vi "verify unique parameter in range - SET.vi"(8 "error in (no error)":errorcluster, 9 "value":dbl, 10 "parameter name":string, 11 "Simulated_CCD_Camera in":refnum<class "Sim_Ixon_Ultra.lvclass">) -> (0 "error out":errorcluster, 3 "Simulated_CCD_Camera out":refnum<class "Sim_Ixon_Ultra.lvclass">)   [LabVIEW 2018, in "Sim_Ixon_Ultra.lvclass"]
uses:
  Sim_Ixon_Ultra.lvclass
  <vilib>/ErrorRing/Error Ring.xnode
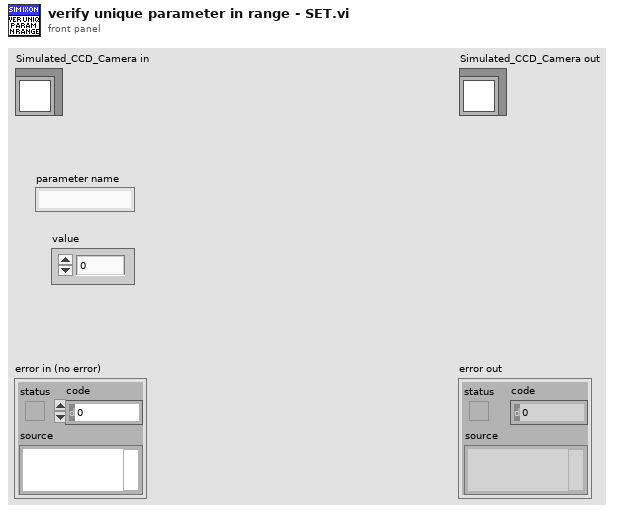
[diagram p1: front panel]
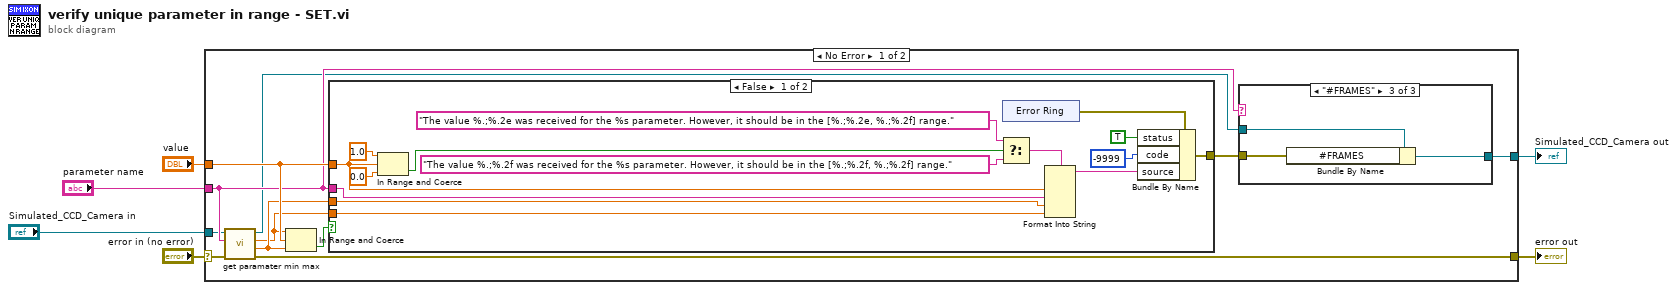
[diagram p0: block diagram]
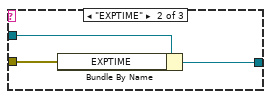
[diagram p3: hidden frame]
diagram:
  n1 = case shown="No Error" "error in (no error)" {
    selector: "error in (no error)" -> [w11 w42]
    tunnel: [w7 w42] -> w5
    tunnel: [w8 w41] -> w4
    tunnel: "Simulated_CCD_Camera in" -> [w12 w41]
    tunnel: "value" -> [w16 _]
    tunnel: "parameter name" -> [w15 _]
    frame No Error {
      n2 = call "get paramater min max.vi"("error in (no error)"=w11, "parameter name"=w15, "Simulated Camera in"=w12) -> ("error out"=w7:errorcluster, "min"=w14:dbl, "max"=w13:dbl, "Simulated Camera out"=w10:refnum<class "Sim_Ixon_Ultra.lvclass">)  [unwired: 5 in]
      n3 = In Range and Coerce(upper limit=w13, x=w16, lower limit=w14) -> (In Range?=w17:bool)  [unwired: 1 out]
      n4 = case shown="False" w17 {
        tunnel: w15 -> [w26 _]
        tunnel: w16 -> [w31 _]
        tunnel: w14 -> [w35 _]
        tunnel: w13 -> [w34 _]
        tunnel: [w25 _] -> w9
        frame False {
          n5 = In Range and Coerce(upper limit=1.0, x=w31, lower limit=0.0 ("upper limit")) -> (In Range?=w30:bool)  [unwired: 1 out]
          n6 = Select(t="The value %.;%.2e was received for the %s parameter. However, it should be in the [%.;%.2e, %.;%.2f] range." ("string"), s=w30, f="The value %.;%.2f was received for the %s parameter. However, it should be in the [%.;%.2f, %.;%.2f] range." ("string")) -> (s? t:f=w27:string)
          n7 = xnode "Error Ring"() -> ("error out"=w39:errorcluster)
          n8 = Format Into String(format string=w27, w31, w26, w35, w34) -> (resulting string=w36:string)  [unwired: 2 in, 1 out]
          n9 = Bundle By Name(cluster=w39, "status"=TRUE, "code"=-9999, "source"=w36) -> (w25:errorcluster)
        }
        frame True {
        }
      }
      n10 = case shown="\"#FRAMES\"" w15 {
        tunnel: w10 -> [w18 w21 w24]
        tunnel: [w18 w20 w23] -> w8
        tunnel: w9 -> [_ w19 w22]
        frame "False", Default {
        }
        frame "EXPTIME" {
          n11 = Bundle By Name(cluster=w21, "EXPTIME"=w19) -> (w20:refnum<class "Sim_Ixon_Ultra.lvclass">)
        }
        frame "#FRAMES" {
          n12 = Bundle By Name(cluster=w24, "#FRAMES"=w22) -> (w23:refnum<class "Sim_Ixon_Ultra.lvclass">)
        }
      }
    }
    frame Error {
    }
  }
  "error out" <- w5
  "Simulated_CCD_Camera out" <- w4
